vi "超标留样全局.vi"() -> ()   [LabVIEW 2016, in "德润DR803L超标留样.lvlib"]
panel:
  out "流程中":bool
  out "超标留样信号":bool
  out "通讯":bool
  out "采样器状态":T1
  in  "当前瓶号":u16
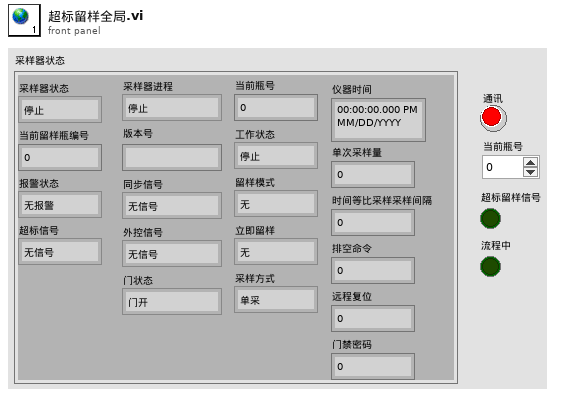
[diagram p1: front panel]
types:
  T1 = cluster{"采样器状态":enum16{"停止", "运行"}, "当前留样瓶编号":u16, "报警状态":enum16{"无报警", "缺水报警"}, "超标信号":enum16{"无信号", "超标信号"}, "采样器进程":enum16{"停止", "待机", "定位校正", "移除瓶盖", "采样瓶排空", "管路润洗", "管存", "进样", "瓶盖密封", "管路排空", "调整采样位置", "采样结束", "采样瓶润洗", "瓶润洗排空"}, "版本号":string, "同步信号":enum16{"无信号", "同步信号"}, "外控信号":enum16{"无信号", "外控信号"}, "门状态":enum16{"门开", "门关"}, "当前瓶号":u16, "工作状态":enum16{"停止", "采样中"}, "留样模式":enum16{"无", "定时留样", "时间等比例", "超标留样", "同步留样", "外控留样"}, "立即留样":enum16{"无", "远程留样"}, "采样方式":enum16{"单采", "双重"}, "仪器时间":timestamp, "单次采样量":u16, "时间等比采样采样间隔":u16, "排空命令":u16, "远程复位":u16, "门禁密码":u16}
diagram:
